vi "Angle Shooter Deck.vi"(8 "reinitialize? (F)":bool, 10 "Shooter Angle":dbl format="%.2f", 11 "Target Angle":dbl) -> (3 "Angle Motor Power Out":dbl)   [LabVIEW 2015]
uses:
  Robot Global Data.vi
  <vilib>/addons/control/pid/pid.llb/PID (DBL).vi
  <vilib>/addons/control/pid/NI_PID_pid.lvlib
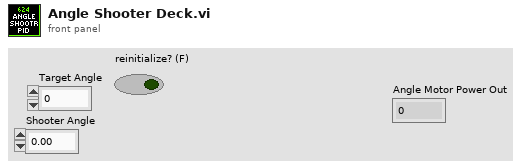
[diagram p1: front panel]
types:
  T1 = typedef "Dashboard Control Data.ctl" = cluster{"Shooter Presets":T2, "Encoder Control":T4, "Steer PID output":cluster{"output high":dbl, "output low":dbl}, " Steer PID gains":cluster{"proportional gain (Kc)":dbl, "integral time (Ti, min)":dbl, "derivative time (Td, min)":dbl}, "Drivetrain Settings":T5, "Vision Packet":T6, "Dashboard Drivetrain Command":T7, "Info/Command Cluster":T9, "Ball Vision Packet":T10, "Intake Presets":T12, "Intake Encoder Control":T14, "Climb Presets":T15, "Goal Output Range":cluster{"output high":dbl, "output low":dbl}, "Enabled Systems":T16, "Auton Presets":T17, "Pressure M":dbl, "Pressure B":dbl}
  T2 = typedef "Shooter Presets.ctl" = cluster{"Batter Shot":T3, "Deep Middle Shot":T3, "Manual Shot":T3, "Left Ticks Per Rotation":dbl, "Right Ticks Per Rotation":dbl, "Low Bar Shot":T3, "Shooter RPM Tolerance":dbl, "IIR Filter Power":dbl, "Trigger Power":dbl, "Fire from Load Delay":i32, "Max Angle":dbl, "Min Angle":dbl, "Angle PID gains":cluster{"P":dbl, "I":dbl, "D":dbl}, "Angle Output":cluster{"output high":dbl, "output low":dbl}, "Shooter Angle Tolerance":dbl, "Vision Shoot x^2":dbl, "Vision Shoot x":dbl, "Axis Camera Offset":dbl, "High Goal Center Height":dbl, "Feed Forward Max Accel":dbl, "Feed Forward Kv":dbl, "Backwards Trigger":dbl, "Shot Finish Delay (ms)":dbl, "Angle Max Current":dbl, "Angle Current Trip Time":dbl, "Intake Angle":dbl, "Vision Shoot c":dbl, "Reset?":bool, "Servo Release Delay":dbl, "Servo Idle Angle":i32, "Servo Hold Angle":i32, "Angle Pot x":dbl, "Angle Pot c":dbl, "Ignore Angle?":bool, "Manual Output?":bool, "Manual Out":dbl, "Max RPM":dbl, "Safty Frist Angle":dbl, "Intake Danger Height":dbl, "Angle Pot B":i32, "Angle Pot M":dbl, "FF Finish RPM":dbl, "RPM PID Right":cluster{"P":dbl, "I":dbl, "D":dbl, "FF":dbl}, "RPM PID Left":cluster{"P":dbl, "I":dbl, "D":dbl, "FF":dbl}, "Backwards RPM":dbl, "Vision RPM":dbl}
  T3 = typedef "Shot Presets.ctl" = cluster{"Left":dbl, "Right":dbl, "Angle":dbl}
  T4 = typedef "Encoder Control.ctl" = cluster{"Right Tick Constant":dbl, "Left Tick Constant":dbl, "Reset?":bool, "Y Dist":cluster{"PID gains":cluster{"proportional gain (Kc)":dbl, "integral time (Ti, min)":dbl, "derivative time (Td, min)":dbl}}, "Y Stop Thresh":dbl, "Y Stop Speed":dbl}
  T5 = typedef "Drivetrain Settings.ctl" = cluster{"Gyro Tolerance":dbl, "Throttle Ramp (ms)":dbl, "Angular rate compensation":bool, "Throttle to Rate Scale":dbl, "Rate compensation gain":dbl, "Kv":dbl, "Ka":dbl, "Feed Forward P":dbl, "Feed Forward D":dbl, "Goal Vision PID gains":cluster{"proportional gain (Kc)":dbl, "integral time (Ti, min)":dbl, "derivative time (Td, min)":dbl}, "Goal Detection Window":dbl, "Creep Rate":dbl}
  T6 = typedef "Goal Vision Packet.ctl" = cluster{"Distance":dbl, "Center X":dbl, "Center Y":dbl, "Found Target?":bool, "Robot Center":dbl, "Angle":dbl}
  T7 = typedef "Dashboard Drivetrain Command.ctl" = cluster{"Drivetrain Vision":T8}
  T8 = typedef "Drivetrain Vision.ctl" = cluster{"Goal Window":dbl, "Ball Window":dbl}
  T9 = typedef "Ball Tracking Command Cluster.ctl" = cluster{"Distance to Ball":dbl, "Desired Angle":dbl, "Command":enum16{"Turn to Ball", "Turn to Angle", "Get Distance"}, "Pixels from Center":dbl}
  T10 = typedef "Ball Vision Packet.ctl" = cluster{"Ball Detected?":bool, "Distance to Ball":dbl, "Desired Angle":dbl, "Pixels from Center":dbl, "Tracking mode":T11}
  T11 = typedef "Tracking Mode.ctl" = enum16{"Turn to Ball", "Turn to Angle"}
  T12 = typedef "Intake Presets.ctl" = cluster{"Intake Speed":dbl, "Outake Speed":dbl, "Low Height":dbl, "Half Height":dbl, "Full Height":dbl, "Angle Speed":dbl, "Angle Tolerance":dbl, "Encoder Scale":dbl, "Load Height":dbl, "Output Range":T13, "Rotation Power Max/Min":dbl, "MaxCurrent":dbl, "Intake Trip Time":dbl, "Idle Height":dbl, "Max Height":dbl, "Reset Encoders?":bool, "PID gains":cluster{"proportional gain (Kc)":dbl, "integral time (Ti, min)":dbl, "derivative time (Td, min)":dbl}}
  T13 = typedef "Drivetrain Output Range.ctl" = cluster{"output high":dbl, "output low":dbl}
  T14 = typedef "IntakeEcoderControl.ctl" = cluster{"Arm Tick Constant":dbl, "Reset?":bool, "Y Dist":cluster{"PID gains":cluster{"proportional gain (Kc)":dbl, "integral time (Ti, min)":dbl, "derivative time (Td, min)":dbl}}, "Y Stop Thresh":dbl, "Y Stop Speed":dbl}
  T15 = typedef "Climb Presets.ctl" = cluster{"Pull Power":dbl, "Time to Hold":dbl, "Extend Power":dbl}
  T16 = typedef "Enabled Systems.ctl" = cluster{"Shoot":bool, "Intake":bool, "DT":bool, "Gyro":bool, "100ms":bool, "US":bool}
  T17 = typedef "Autonomous Presets.ctl" = cluster{"Pitch Limit":dbl, "Roll Limit":dbl, "Ultrasonic Limit":dbl, "Start Position":dbl, "Cross Position":dbl}
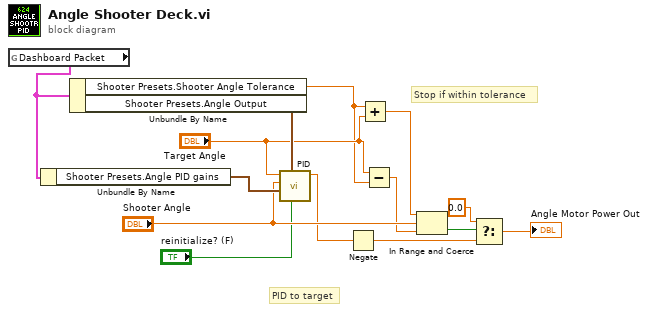
[diagram p0: block diagram]
diagram:
  # "Stop if within tolerance"
  # "PID to target"
  n1 = global read "Robot Global Data.vi" "Dashboard Packet"() -> (w13:T1)
  n2 = Unbundle By Name(w13) -> ("Shooter Presets.Angle PID gains"=w14:cluster{"P":dbl, "I":dbl, "D":dbl})
  n3 = Unbundle By Name(w13) -> ("Shooter Presets.Shooter Angle Tolerance"=w8:dbl, "Shooter Presets.Angle Output"=w12:cluster{"output high":dbl, "output low":dbl})
  n4 = call-poly <vilib>:"PID.vi"("reinitialize? (F)"="reinitialize? (F)", "output range"=w12, "PID gains"=w14, "process variable"="Shooter Angle", "setpoint"="Target Angle") -> ("output"=w2:dbl)  [unwired: 5 in, 1 out]
  n5 = Negate(x=w2) -> (-x=w1:dbl)
  n6 = Add(x=w8, y="Target Angle") -> (x+y=w10:dbl)
  n7 = Subtract(x="Target Angle", y=w8) -> (x-y=w7:dbl)
  n8 = In Range and Coerce(upper limit=w10, x="Shooter Angle", lower limit=w7) -> (In Range?=w6:bool)  [unwired: 1 out]
  n9 = Select(t=0.0, s=w6, f=w1) -> (s? t:f=→"Angle Motor Power Out":dbl)
